vi "tq_rpm_to_kw_hp.vi"(10 "RPM":dbl, 11 "Torque":dbl) -> (2 "hp":dbl, 3 "kw":dbl)   [LabVIEW 2014]
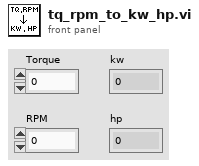
[diagram p1: front panel]
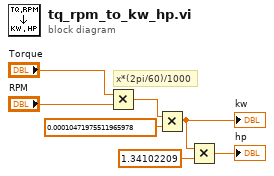
[diagram p0: block diagram]
diagram:
  # "x*(2pi/60)/1000"
  n1 = Multiply(x="Torque", y="RPM") -> (x*y=w3:dbl)
  n2 = Multiply(x=w3, y=0.00010471975511965978) -> (x*y=w2:dbl)
  "kw" <- w2
  n3 = Multiply(x=w2, y=1.34102209) -> (x*y=→"hp":dbl)
